vi "Propeller.vi"() -> ()   [LabVIEW 2011]
panel:
  in  "Propeller":dbl
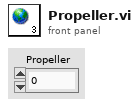
[diagram p1: front panel]
diagram:
